vi "Tree Destroy.vi"(8 "error in (no error)":errorcluster, 11 "Tree DVR in":refnum<data-value>) -> (0 "error out":errorcluster)   [LabVIEW 2013, in "MDSplus.lvlib"]
uses:
  <vilib>/MDSplus/Library/MDSplus.lvlib
  <vilib>/MDSplus/Classes/Tree_Class/Tree.lvclass
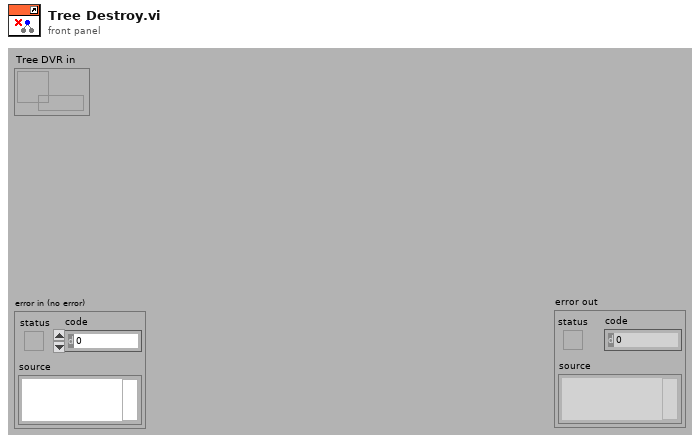
[diagram p1: front panel]
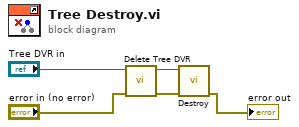
[diagram p0: block diagram]
diagram:
  n1 = call <vilib>:"Delete Tree DVR.vi"("error in (no error)"="error in (no error)", "Tree DVR in"="Tree DVR in") -> ("error out"=w2:errorcluster, "Tree out"=w3:refnum<class "Tree.lvclass">)  [unwired: 8 in]
  n2 = call-dynamic "Destroy.vi"("error in (no error)"=w2, "Tree in"=w3) -> ("error out"=→"error out":errorcluster)  [unwired: 9 in]
